vi "ConversorGradosCF.vi"(11 "GradosC":dbl) -> (2 "Grados F":dbl, 3 "Grados C":dbl)   [LabVIEW 2019]
doc: "Convierte la temperatura de grados centigrados a grados Fahrenheit."
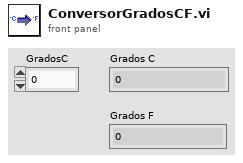
[diagram p1: front panel]
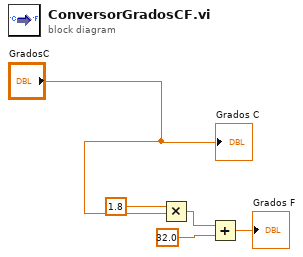
[diagram p0: block diagram]
diagram:
  n1 = Multiply(x=1.8, y="GradosC") -> (x*y=w3:dbl)
  n2 = Add(x=w3, y=32.0) -> (x+y=→"Grados F":dbl)
  "Grados C" <- "GradosC"
